vi "Mark All Temp Variables as Permanent.vi"(8 "error in (no error)":errorcluster, 9 "SyncRef?(F)":bool, 10 "Path":path, 11 "CSM-Static-Variable-Manager in":refnum<class "CSM-Static-Variable-Manager.lvclass">) -> (0 "error out":errorcluster, 3 "CSM-Static-Variable-Manager out":refnum<class "CSM-Static-Variable-Manager.lvclass">)   [LabVIEW 2017, in "INI-Static-Variable-Support.lvlib" / "CSM-Static-Variable-Manager.lvclass"]
uses:
  CSM-Static-Variable-Manager.lvclass
  CSM-Static-Variable-Manager.lvclass/CSM-Static-Variable-Manager.ctl
  LabVIEW-Config/Config.ctl
  LabVIEW-Config/LineToken.ctl
  LabVIEW-Config/LabVIEW-Config.lvlib
  INI-Static-Variable-Support.lvlib
  <userlib>/_NEVSTOP/Communicable State Machine(CSM)/Communicable State Machine.lvlib
  <userlib>/_NEVSTOP/Communicable State Machine(CSM)/addons/API-String-Arugments-Support/API String Arguments Support.lvlib
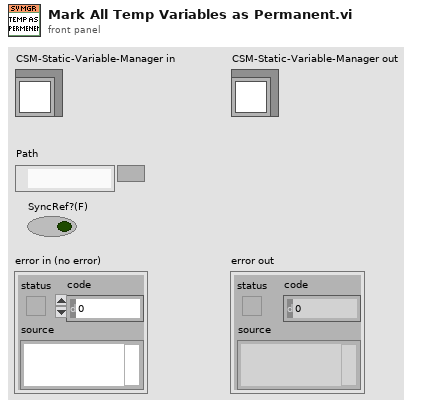
[diagram p1: front panel]
types:
  T1 = typedef "LabVIEW-Config.lvlib/Config.ctl" = cluster{"Path":path, "Lines":string[], "Tokens":T2[], "Modified?":bool}
  T2 = typedef "LabVIEW-Config.lvlib/LineToken.ctl" = enum8{"comment", "section", "key", "more"}
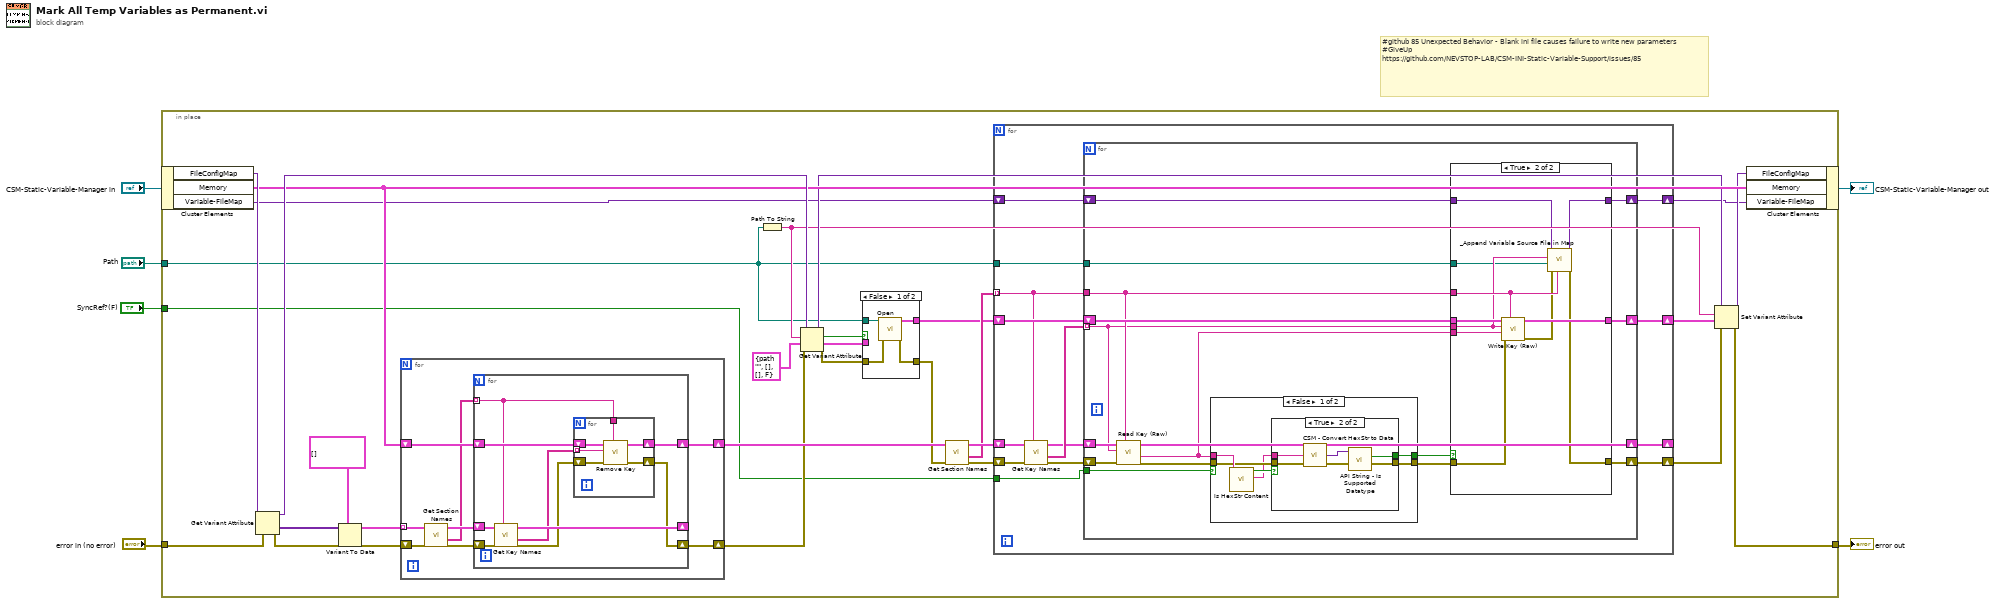
[diagram p0: block diagram]
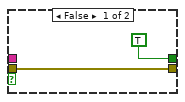
[diagram p4: hidden frame]
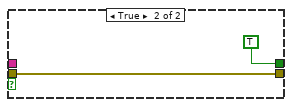
[diagram p5: hidden frame]
diagram:
  # "#github 85 Unexpected Behavior - Blank ini file causes failure to write new parameters #GiveUp\nhttps://github.com/NEVSTOP-LAB/CSM-INI-Static-Variable-Support/issues/85"
  n1 = in-place {
    in-place-border: "error in (no error)" -> [w33]
    in-place-border: [w16] -> w3
    in-place-border: "Path" -> [w8]
    in-place-border: "SyncRef?(F)" -> [w10]
    n2 = in-place-cluster #1("CSM-Static-Variable-Manager in") -> ("FileConfigMap"=w36:variant, "Memory"=w28:T1, "Variable-FileMap"=w9:variant)
    n3 = Get Variant Attribute(Variant=w36, error in=w33) -> (duplicate Variant=w29:variant, values=w35:variant[], error out=w34:errorcluster)  [unwired: 2 in, 1 out]
    n4 = Variant To Data(error in=w34, type=T1[] [], Variant=w35) -> (data=w30:T1[], error out=w32:errorcluster)
    n5 = for {
      shift-right: [w108] -> w27
      shift-left: w28 -> [w109]
      shift-right: [w103] -> w22
      shift-left: w32 -> [w106]
      tunnel: w30 -> [w110] mode=indexing
      n6 = call "Get Section Names.vi"("error in (no error)"=w106, "Config in"=w110) -> ("error out"=w105:errorcluster, "Section Names"=w104:string[], "Config out"=w107:T1)  [unwired: 7 in]
      n7 = for {
        shift-right: [w115] -> w108
        shift-left: w109 -> [w116]
        shift-right: [w112] -> w103
        shift-left: w105 -> [w117]
        tunnel: w104 -> [w114] mode=indexing
        shift-right: [w119] -> _
        shift-left: w107 -> [w118]
        n8 = call "Get Key Names.vi"("Section Name"=w114, "error in (no error)"=w117, "Config in"=w118) -> ("error out"=w113:errorcluster, "Key Names"=w111:string[], "Config out"=w119:T1)  [unwired: 5 in, 1 out]
        n9 = for {
          tunnel: w114 -> [w123]
          tunnel: w111 -> [w120] mode=indexing
          shift-right: [w124] -> w115
          shift-left: w116 -> [w125]
          shift-right: [w121] -> w112
          shift-left: w113 -> [w122]
          n10 = call "Remove Key.vi"("Section Name"=w123, "error in (no error)"=w122, "Key Name"=w120, "Config in"=w125) -> ("error out"=w121:errorcluster, "Config out"=w124:T1)  [unwired: 5 in, 1 out]
        }
      }
    }
    n11 = Path To String(path=w8) -> (string=w19:string)
    n12 = Get Variant Attribute(Variant=w29, name=w19, default value (empty Variant)=T1 {"Path"=path "", "Lines"=[], "Tokens"=[], "Modified?"=FALSE} ("Config out"), error in=w22) -> (duplicate Variant=w23:variant, found=w12:bool, value=w11:T1, error out=w13:errorcluster)
    n13 = case shown="False" w12 {
      tunnel: w8 -> [w40 _]
      tunnel: [w39 w41] -> w15
      tunnel: [w38 w42] -> w14
      tunnel: w13 -> [w37 w42]
      tunnel: w11 -> [_ w41]
      frame False {
        n14 = call "Open.vi"("error in (no error)"=w37, "Path"=w40) -> ("error out"=w38:errorcluster, "Config"=w39:T1)  [unwired: 6 in, 2 out]
      }
      frame True {
      }
    }
    n15 = call "Get Section Names.vi"("error in (no error)"=w14, "Config in"=w27) -> ("error out"=w25:errorcluster, "Section Names"=w24:string[], "Config out"=w26:T1)  [unwired: 7 in]
    n16 = for {
      shift-right: [w50] -> w17
      shift-left: w25 -> [w55]
      tunnel: w24 -> [w53] mode=indexing
      shift-right: [w49] -> _
      shift-left: w26 -> [w56]
      shift-right: [w47] -> w18
      shift-left: w15 -> [w54]
      tunnel: w10 -> [w46]
      shift-right: [w43] -> w7
      shift-left: w9 -> [w45]
      tunnel: w8 -> [w44]
      n17 = call "Get Key Names.vi"("Section Name"=w53, "error in (no error)"=w55, "Config in"=w56) -> ("error out"=w51:errorcluster, "Key Names"=w52:string[], "Config out"=w48:T1)  [unwired: 5 in, 1 out]
      n18 = for {
        tunnel: w53 -> [w67]
        tunnel: w52 -> [w66] mode=indexing
        shift-right: [w71] -> w50
        shift-left: w51 -> [w70]
        shift-right: [w69] -> w49
        shift-left: w48 -> [w68]
        shift-right: [w65] -> w47
        shift-left: w54 -> [w72]
        tunnel: w46 -> [w60]
        shift-right: [w57] -> w43
        shift-left: w45 -> [w58]
        tunnel: w44 -> [w59]
        n19 = call "Read Key (Raw).vi"("Section Name"=w67, "error in (no error)"=w70, "Key Name"=w66, "Config in"=w68) -> ("error out"=w64:errorcluster, "Content"=w62:string, "Config out"=w69:T1)  [unwired: 4 in, 1 out]
        n20 = case shown="False" w60 {
          tunnel: w62 -> [w92 _]
          tunnel: [w88 TRUE ("HexStr Content")] -> w61
          tunnel: w64 -> [w91 w101]
          tunnel: [w90 w101] -> w63
          frame False {
            n21 = call "Is HexStr Content.vi"("Content"=w92) -> ("hexStr"=w87:string, "HexStr Content"=w89:bool)  [unwired: 9 in]
            n22 = case shown="True" w89 {
              tunnel: w87 -> [_ w100]
              tunnel: w91 -> [w93 w99]
              tunnel: [w93 w96] -> w90
              tunnel: [TRUE ("HexStr Content") w95] -> w88
              frame False {
              }
              frame True {
                n23 = call <userlib>:"CSM - Convert HexStr to Data.vi"("HEX String"=w100, "error in (no error)"=w99) -> ("Variant"=w98:variant, "error out"=w97:errorcluster)  [unwired: 6 in]
                n24 = call <userlib>:"API String - Is Supported Datatype.vi"("error in (no error)"=w97, "data"=w98) -> ("error out"=w96:errorcluster, "supported datatype?"=w95:bool)  [unwired: 7 in, 1 out]
              }
            }
          }
          frame True {
          }
        }
        n25 = case shown="True" w61 {
          tunnel: w72 -> [w74 w86]
          tunnel: [w75 w80] -> w71
          tunnel: w67 -> [_ w82]
          tunnel: w66 -> [_ w79]
          tunnel: [w74 w85] -> w65
          tunnel: w63 -> [w75 w84]
          tunnel: w62 -> [_ w83]
          tunnel: w59 -> [_ w78]
          tunnel: w58 -> [w73 w77]
          tunnel: [w73 w76] -> w57
          frame False {
          }
          frame True {
            n26 = call "Write Key (Raw).vi"("Section Name"=w82, "error in (no error)"=w84, "Content"=w83, "Key Name"=w79, "Config in"=w86) -> ("error out"=w81:errorcluster, "Config out"=w85:T1)  [unwired: 4 in, 1 out]
            n27 = call "_Append Variable Source File in Map.vi"("String"=w82, "error in (no error)"=w81, "dup path"=w78, "Content"=w79, "Variable-FileMap"=w77) -> ("error out"=w80:errorcluster, "Variant"=w76:variant)  [unwired: 5 in]
          }
        }
      }
    }
    n28 = Set Variant Attribute(Variant=w23, name=w19, value=w18, error in=w17) -> (Variant out=w20:variant, error out=w16:errorcluster)  [unwired: 1 out]
    n29 = in-place-cluster #1("FileConfigMap"=w20, "Memory"=w28, "Variable-FileMap"=w7) -> (→"CSM-Static-Variable-Manager out":refnum<class "CSM-Static-Variable-Manager.lvclass">)
  }
  "error out" <- w3
